vi "FormatStringTime.vi"(10 "TimeZone":T1, 11 "Format String":string="%<%H:%M:%S>T") -> (3 "Format String":string)   [LabVIEW 2021, in "RocketPlot.lvlib"]
uses:
  RocketPlot.lvlib
  TypeDefs/TimeZone.ctl
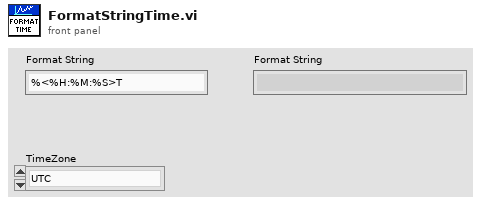
[diagram p1: front panel]
types:
  T1 = typedef "RocketPlot.lvlib/TimeZone.ctl" = enum16{"UTC", "Local"}
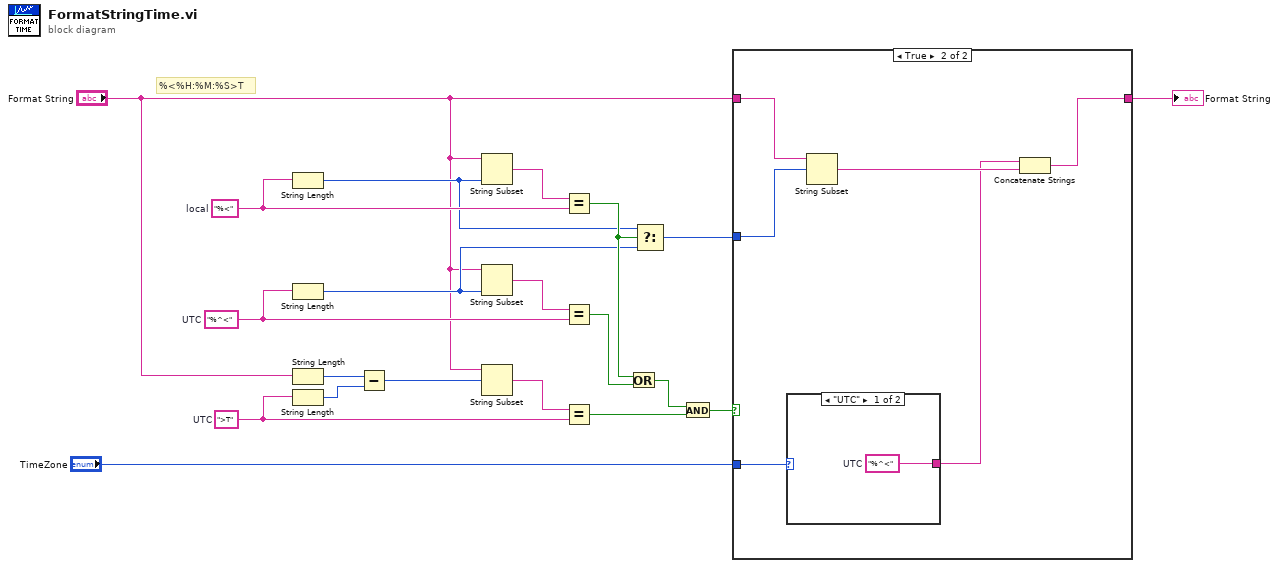
[diagram p0: block diagram]
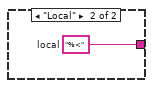
[diagram p3: hidden frame]
diagram:
  w15 = ">T"  # UTC
  w18 = "%^<"  # UTC
  w19 = "%<"  # local
  # "%<%H:%M:%S>T"
  n1 = String Length(string=w19) -> (length=w5:i32)
  n2 = String Length(string=w18) -> (length=w4:i32)
  n3 = String Length(string="Format String") -> (length=w14:i32)
  n4 = String Length(string=w15) -> (length=w13:i32)
  n5 = Subtract(x=w14, y=w13) -> (x-y=w12:i32)
  n6 = String Subset(string="Format String", length (rest)=w5) -> (substring=w20:string)  [unwired: 1 in]
  n7 = String Subset(string="Format String", length (rest)=w4) -> (substring=w17:string)  [unwired: 1 in]
  n8 = String Subset(string="Format String", offset (0)=w12) -> (substring=w16:string)  [unwired: 1 in]
  n9 = Equal?(x=w20, y=w19) -> (x = y?=w6:bool)
  n10 = Equal?(x=w17, y=w18) -> (x = y?=w7:bool)
  n11 = Equal?(x=w16, y=w15) -> (x = y?=w10:bool)
  n12 = Or(x=w6, y=w7) -> (x .or. y?=w11:bool)
  n13 = Select(t=w5, s=w6, f=w4) -> (s? t:f=w3:i32)
  n14 = And(x=w11, y=w10) -> (x .and. y?=w9:bool)
  n15 = case shown="True" w9 {
    tunnel: "Format String" -> [w21 w27]
    tunnel: [w21 w22] -> w2
    tunnel: "TimeZone" -> [_ w24]
    tunnel: w3 -> [_ w26]
    frame False {
    }
    frame True {
      n16 = case shown="\"UTC\"" w24 {
        tunnel: [w28 w29] -> w23
        frame "UTC" {
          w28 = "%^<"  # UTC
        }
        frame "Local" {
          w29 = "%<"  # local
        }
      }
      n17 = String Subset(string=w27, offset (0)=w26) -> (substring=w25:string)  [unwired: 1 in]
      n18 = Concatenate Strings(w23, w25) -> (w22:string)
    }
  }
  "Format String" <- w2
